vi "TOP-串口通信模块.vi"(8 "错误输入（无错误）":errorcluster, 11 "串口模块输入":T1) -> (0 "error out":errorcluster, 3 "数据输出":variant)   [LabVIEW 2017]
uses:
  be20d104-bee2-4132-b2b8-f45edb506baf.vi
  30f28544-4a48-4f37-80c2-698119a7172f.vi
  <vilib>/Instr/_visa.llb/VISA Configure Serial Port (Instr).vi
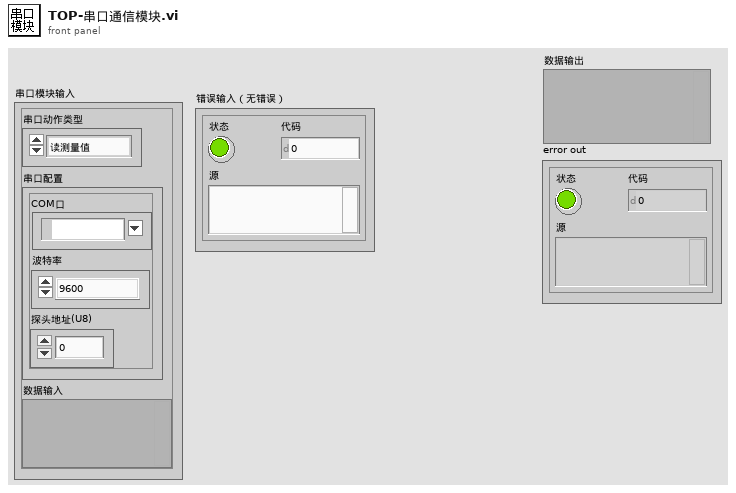
[diagram p1: front panel]
types:
  T1 = typedef "串口模块输入.ctl" = cluster{"串口动作类型":T2, "串口配置":T3, "数据输入":variant}
  T2 = typedef "串口动作类型.ctl" = enum16{"读测量值", "设置报警值", "设置地址", "设置系数", "广播修改波特率", "关闭串口"}
  T3 = typedef "串口配置.ctl" = cluster{"COM口":refnum<visa-resource-name>, "波特率":enum16{"9600", "19200"}, "探头地址(U8)":u8}
  T4 = typedef "测量值读取.ctl" = cluster{"测量值":dbl, "CRC":bool, "接收指令":string}
  T5 = typedef "探头系数.ctl" = cluster{"N1":u16, "N2":u16}
  T6 = typedef "簇-输入.ctl" = cluster{"配置文件动作":T7, "数据输入":variant}
  T7 = typedef "枚举-配置文件动作.ctl" = enum16{"初始化加载配置", "读取配置", "写入-屏幕键盘", "写入-静音延迟", "写入-主要探头类型", "写入-串口配置", "写入-累积定时", "写入-导出定时", "保存配置到文件"}
  T8 = typedef "簇-配置文件内容.ctl" = cluster{"调试模式？":bool, "屏幕键盘？":bool, "软件版本":string, "静音延迟 s":u16, "主要探头类型":T9, "串口配置":cluster{"COM口":refnum<visa-resource-name>, "波特率":enum16{"9600", "19200"}, "读写超时ms":i16, "丢包判定次数":i16}, "定时配置-累积分段":T10, "定时配置-自动导出":cluster{"定时配置-自动导出":T10, "分别导出?":bool}}
  T9 = typedef "枚举-主要探头类型.ctl" = enum16{"网络探头", "串口探头"}
  T10 = typedef "簇-定时配置.ctl" = cluster{"定时模式":enum16{"绝对时间", "相对时间"}, "单位":enum16{"年", "月", "日", "时", "分"}, "间隔":u8, "目标时刻":timestamp}
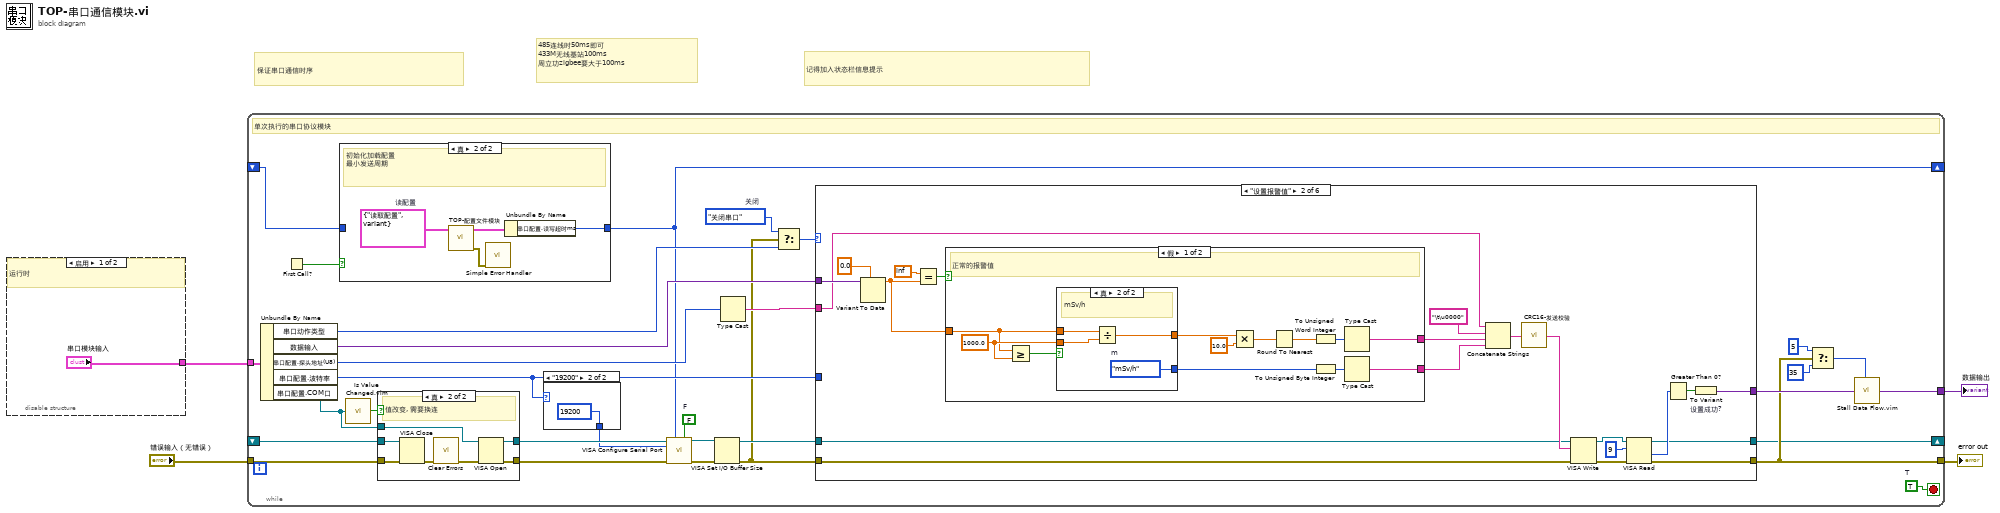
[diagram p0: block diagram]
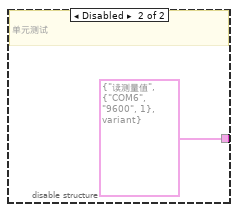
[diagram p2: hidden frame]
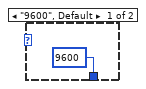
[diagram p5: hidden frame]
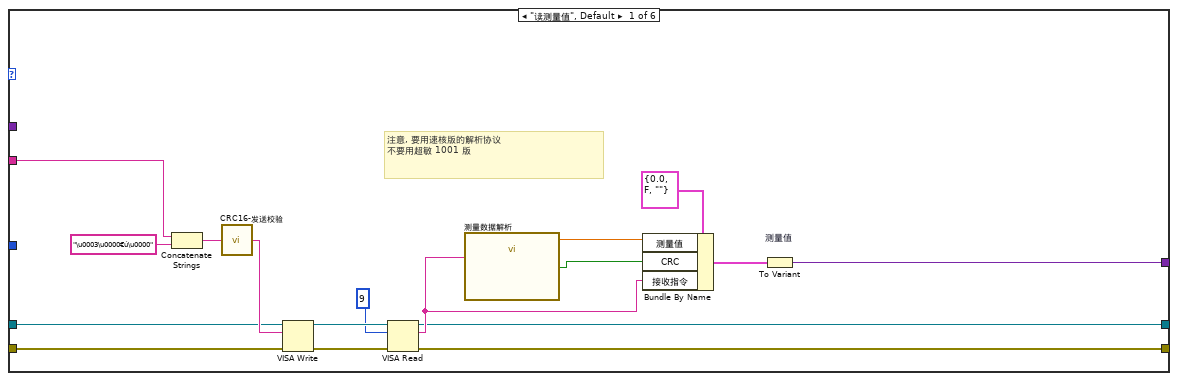
[diagram p6: hidden frame]
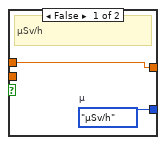
[diagram p7: hidden frame]
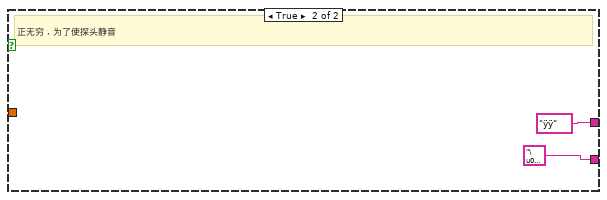
[diagram p8: hidden frame]
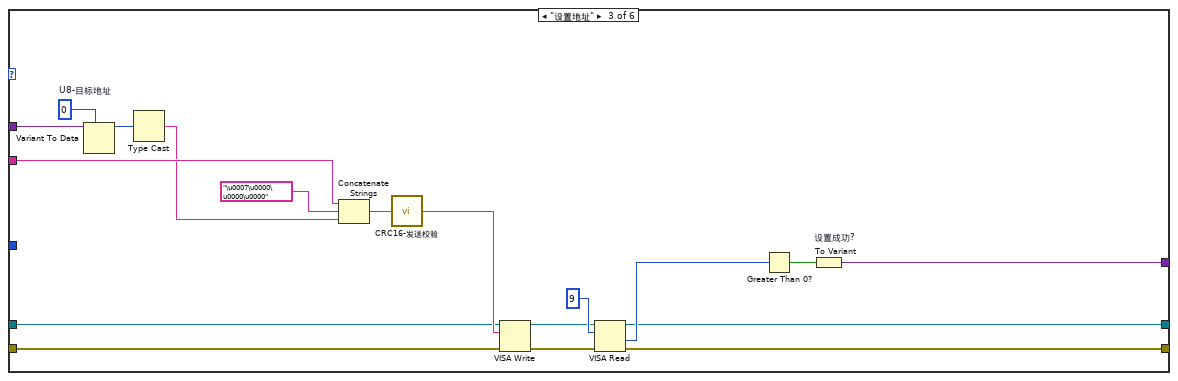
[diagram p9: hidden frame]
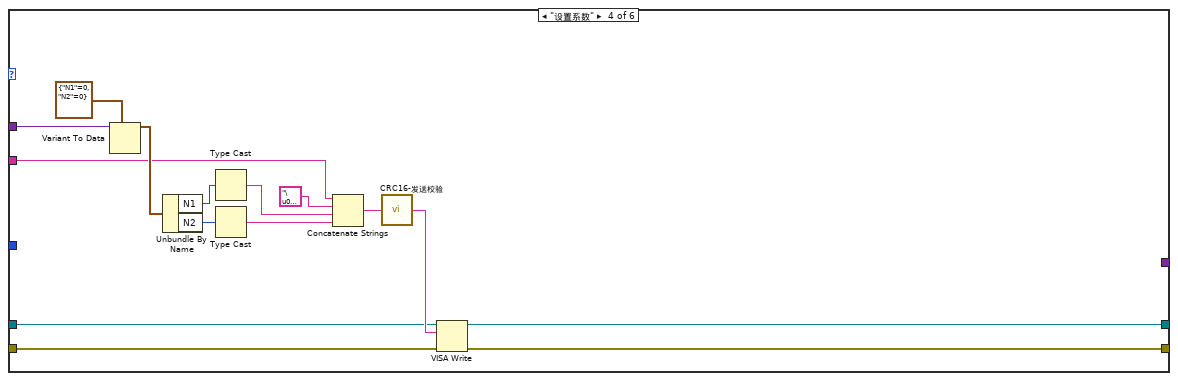
[diagram p10: hidden frame]
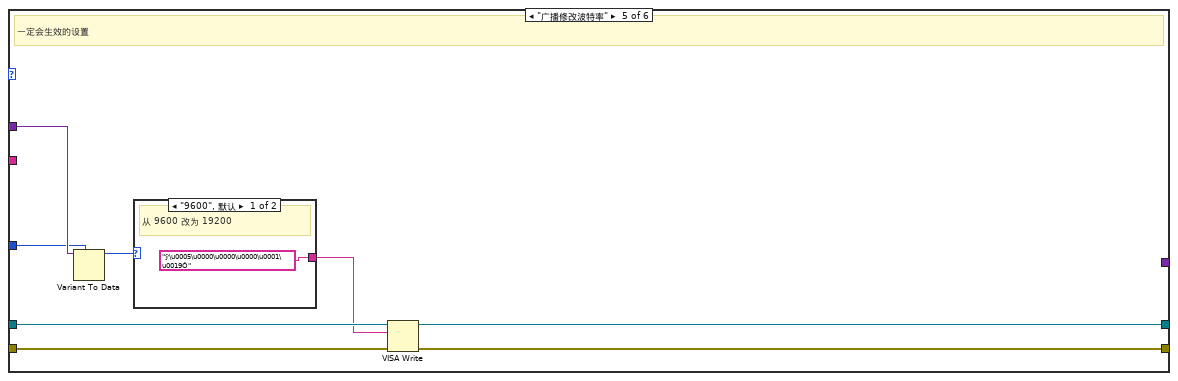
[diagram p11: hidden frame]
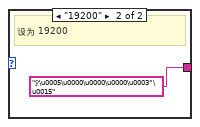
[diagram p12: hidden frame]
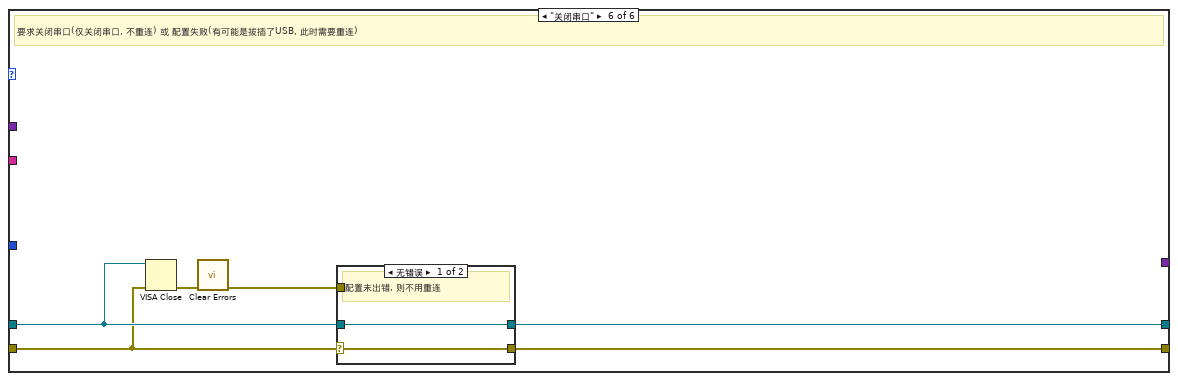
[diagram p13: hidden frame]
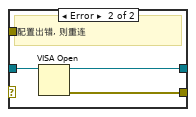
[diagram p14: hidden frame]
diagram:
  # "485连线时50ms即可\n433M无线基站100ms\n周立功zigbee要大于100ms"
  # "记得加入状态栏信息提示"
  # "保证串口通信时序"
  n1 = disable-structure shown="启用" {
    disable-tunnel: ["串口模块输入" T1 {"串口动作类型"=enum."读测量值", "串口配置"={"COM口"="COM6", "波特率"=enum."9600", "探头地址(U8)"=1}, "数据输入"=variant} ("串口模块输入")] -> w4
    frame Enabled {
      # "运行时"
    }
    frame Disabled {
      # "单元测试"
    }
  }
  n2 = while {
    tunnel: w4 -> [w36]
    tunnel: [w18] -> w3
    tunnel: "错误输入（无错误）" -> [w23]
    tunnel: [w17] -> w1
    shift-right: [w13] -> _
    shift-left: _ -> [w11]
    shift-right: [w8] -> _
    shift-left: _ -> [w7]
    stop <- w37 stop-if-true
    w22 = 串口动作类型."关闭串口"  # 关闭
    w31 = FALSE  # F
    w37 = TRUE  # T
    # "单次执行的串口协议模块"
    n3 = Unbundle By Name(w36) -> ("串口动作类型"=w21:T2, "数据输入"=w26:variant, "串口配置.探头地址(U8)"=w27:u8, "串口配置.波特率"=w25:enum16{"9600", "19200"}, "串口配置.COM口"=w12:refnum<visa-resource-name>)
    n4 = First Call?() -> (First Call?: T/F=w9:bool)
    n5 = case shown="真" w9 {
      tunnel: [w38 w39] -> w8
      tunnel: w7 -> [w38 _]
      frame False {
      }
      frame True {
        w42 = T6 {"配置文件动作"=enum."读取配置", "数据输入"=variant}  # 读配置
        # "初始化加载配置\n最小发送周期"
        n6 = call "TOP-配置文件模块.vi"("输入"=w42) -> ("error out"=w41:errorcluster, "配置文件"=w40:T8)  [unwired: 9 in]
        n7 = call <vilib>:"Simple Error Handler.vi"("error in (no error)"=w41) -> ()  [unwired: 4 in, 5 out]
        n8 = Unbundle By Name(w40) -> ("串口配置.读写超时ms"=w39:i16)
      }
    }
    n9 = call "Is Value Changed.vim"("value"=w12) -> ("changed or first call?"=w19:bool)
    n10 = case shown="真" w19 {
      tunnel: [w43 w51] -> w33
      tunnel: [w44 w50] -> w32
      tunnel: w23 -> [w43 w49]
      tunnel: w11 -> [w44 w45]
      tunnel: w12 -> [_ w46]
      frame False {
        # "值未变, 不用重连"
      }
      frame True {
        # "值改变, 需要换连"
        n11 = VISA Close(VISA resource name=w45, error in (no error)=w49) -> (error out=w48:errorcluster)
        n12 = call <vilib>:"Clear Errors.vi"("error in (no error)"=w48) -> ("error out"=w47:errorcluster)  [unwired: 5 in, 1 out]
        n13 = VISA Open(error in (no error)=w47, VISA resource name=w46) -> (VISA resource name=w50:refnum<visa-resource-name>, error out=w51:errorcluster)  [unwired: 3 out]
      }
    }
    n14 = case shown="\"19200\"" w25 {
      tunnel: [u32 9600 ("baud rate (9600)") u32 19200 ("baud rate (9600)")] -> w24
      frame "9600", Default {
      }
      frame "19200" {
      }
    }
    n15 = call-poly "VISA Configure Serial Port"("VISA resource name"=w32, "timeout (10sec)"=w8, "Enable Termination\nChar (T)"=w31, "baud rate (9600)"=w24, "error in (no error)"=w33) -> ("VISA resource name out"=w34:refnum<visa-resource-name>, "error out"=w35:errorcluster)  [unwired: 3 in, 6 out]
    n16 = VISA Set I/O Buffer Size(VISA resource name=w34, error in (no error)=w35) -> (VISA resource name out=w30:refnum<visa-resource-name>, error out=w10:errorcluster)  [unwired: 2 out]
    n17 = Type Cast(x=w27) -> (*(type *) &x=w29:string)  [unwired: 1 in]
    n18 = Select(t=w22, s=w10, f=w21) -> (s? t:f=w20:T2)
    n19 = case shown="\"设置报警值\"" w20 {
      tunnel: w26 -> [_ w85 w129 w144 w148 _]
      tunnel: w30 -> [w64 w80 w118 w133 w152 w159]
      tunnel: w29 -> [w63 w82 w125 w135 _ _]
      tunnel: [w62 w74 w115 _ _ _] -> w28
      tunnel: w25 -> [_ _ _ _ w147 _]
      tunnel: w10 -> [w61 w73 w113 w132 w150 w156]
      tunnel: [w60 w72 w114 w131 w149 w158] -> w17
      tunnel: [w54 w71 w112 w130 w145 w157] -> w13
      frame "读测量值", Default {
        # "注意, 要用速核版的解析协议\n不要用超敏 1001 版"
        n20 = Concatenate Strings(w63, "\u0003\u0000€ú\u0000") -> (w70:string)
        n21 = call "CRC16-发送校验.vi"("净数据"=w70) -> ("完整输出"=w65:string)
        n22 = VISA Write(VISA resource name=w64, write buffer=w65, error in (no error)=w61) -> (VISA resource name out=w67:refnum<visa-resource-name>, error out=w68:errorcluster)  [unwired: 1 out]
        n23 = VISA Read(VISA resource name=w67, byte count=u32 9 ("字节总数"), error in (no error)=w68) -> (VISA resource name out=w54:refnum<visa-resource-name>, read buffer=w55:string, error out=w60:errorcluster)  [unwired: 1 out]
        n24 = call "测量数据解析.vi"("完整输入"=w55) -> ("CRC？"=w58:bool, "测量值"=w57:dbl)  [unwired: 8 in, 1 out]
        n25 = Bundle By Name(cluster=T4 {"测量值"=0.0, "CRC"=FALSE, "接收指令"=""} ("测量值读取"), "测量值"=w57, "CRC"=w58, "接收指令"=w55) -> (w56:T4)
        n26 = To Variant "测量值"(anything=w56) -> (Variant=w62:variant)
      }
      frame "设置报警值" {
        n27 = Variant To Data(type=0.0, Variant=w85) -> (data=w83:dbl)  [unwired: 1 in, 1 out]
        n28 = Equal?(x=inf, y=w83) -> (x = y?=w91:bool)
        n29 = case shown="假" w91 {
          tunnel: [w94 "\u0001"] -> w88
          tunnel: [w93 "ÿÿ"] -> w89
          tunnel: w83 -> [w92 _]
          frame False {
            w102 = 1000.0 ("y")
            # "正常的报警值"
            n30 = Greater Or Equal?(x=w92, y=w102) -> (x >= y?=w103:bool)
            n31 = case shown="真" w103 {
              tunnel: w92 -> [w104 w108]
              tunnel: [w105 w109] -> w96
              tunnel: w102 -> [_ w107]
              tunnel: [w104 w106] -> w101
              frame False {
                w105 = enum8{"μSv/h", "mSv/h"}."μSv/h"  # μ
                # "μSv/h"
              }
              frame True {
                w109 = enum8{"μSv/h", "mSv/h"}."mSv/h"  # m
                # "mSv/h"
                n32 = Divide(x=w108, y=w107) -> (x/y=w106:dbl)
              }
            }
            n33 = Multiply(x=w101, y=10.0) -> (x*y=w98:dbl)
            n34 = Round To Nearest(number=w98) -> (nearest integer value=w97:dbl)
            n35 = To Unsigned Word Integer(number=w97) -> (unsigned 16bit integer=w99:u16)
            n36 = To Unsigned Byte Integer(number=w96) -> (unsigned 8bit integer=w95:u8)
            n37 = Type Cast(x=w99) -> (*(type *) &x=w93:string)  [unwired: 1 in]
            n38 = Type Cast(x=w95) -> (*(type *) &x=w94:string)  [unwired: 1 in]
          }
          frame True {
            # "正无穷 , 为了使探头静音"
          }
        }
        n39 = Concatenate Strings(w82, "\t\u0000", w89, w88) -> (w87:string)
        n40 = call "CRC16-发送校验.vi"("净数据"=w87) -> ("完整输出"=w81:string)
        n41 = VISA Write(VISA resource name=w80, write buffer=w81, error in (no error)=w73) -> (VISA resource name out=w79:refnum<visa-resource-name>, error out=w76:errorcluster)  [unwired: 1 out]
        n42 = VISA Read(VISA resource name=w79, byte count=u32 9 ("字节总数"), error in (no error)=w76) -> (VISA resource name out=w71:refnum<visa-resource-name>, return count=w77:u32, error out=w72:errorcluster)  [unwired: 1 out]
        n43 = Greater Than 0?(x=w77) -> (x > 0?=w75:bool)
        n44 = To Variant "设置成功?"(anything=w75) -> (Variant=w74:variant)
      }
      frame "设置地址" {
        w128 = u8 0  # U8-目标地址
        n45 = Variant To Data(type=w128, Variant=w129) -> (data=w127:u8)  [unwired: 1 in, 1 out]
        n46 = Type Cast(x=w127) -> (*(type *) &x=w124:string)  [unwired: 1 in]
        n47 = Concatenate Strings(w125, "\u0007\u0000\u0000\u0000", w124) -> (w123:string)
        n48 = call "CRC16-发送校验.vi"("净数据"=w123) -> ("完整输出"=w119:string)
        n49 = VISA Write(VISA resource name=w118, write buffer=w119, error in (no error)=w113) -> (VISA resource name out=w120:refnum<visa-resource-name>, error out=w122:errorcluster)  [unwired: 1 out]
        n50 = VISA Read(VISA resource name=w120, byte count=u32 9 ("字节总数"), error in (no error)=w122) -> (VISA resource name out=w112:refnum<visa-resource-name>, return count=w117:u32, error out=w114:errorcluster)  [unwired: 1 out]
        n51 = Greater Than 0?(x=w117) -> (x > 0?=w116:bool)
        n52 = To Variant "设置成功?"(anything=w116) -> (Variant=w115:variant)
      }
      frame "设置系数" {
        n53 = Variant To Data(type=T5 {"N1"=0, "N2"=0}, Variant=w144) -> (data=w142:T5)  [unwired: 1 in, 1 out]
        n54 = Unbundle By Name(w142) -> ("N1"=w137:u16, "N2"=w136:u16)
        n55 = Type Cast(x=w137) -> (*(type *) &x=w138:string)  [unwired: 1 in]
        n56 = Type Cast(x=w136) -> (*(type *) &x=w140:string)  [unwired: 1 in]
        n57 = Concatenate Strings(w135, "\u0012", w138, w140) -> (w141:string)
        n58 = call "CRC16-发送校验.vi"("净数据"=w141) -> ("完整输出"=w134:string)
        n59 = VISA Write(VISA resource name=w133, write buffer=w134, error in (no error)=w132) -> (VISA resource name out=w130:refnum<visa-resource-name>, error out=w131:errorcluster)  [unwired: 1 out]
      }
      frame "广播修改波特率" {
        # "一定会生效的设置"
        n60 = Variant To Data(type=w147, Variant=w148) -> (data=w146:enum16{"9600", "19200"})  [unwired: 1 in, 1 out]
        n61 = case shown="\"9600\", 默认" w146 {
          tunnel: ["ÿ\u0005\u0000\u0000\u0000\u0001\u0019Ô" "ÿ\u0005\u0000\u0000\u0000\u0003˜\u0015"] -> w151
          frame "9600", Default {
            # "从 9600 改为 19200"
          }
          frame "19200" {
            # "设为 19200"
          }
        }
        n62 = VISA Write(VISA resource name=w152, write buffer=w151, error in (no error)=w150) -> (VISA resource name out=w145:refnum<visa-resource-name>, error out=w149:errorcluster)  [unwired: 1 out]
      }
      frame "关闭串口" {
        # "要求关闭串口(仅关闭串口, 不重连) 或 配置失败(有可能是拔插了USB, 此时需要重连)"
        n63 = VISA Close(VISA resource name=w159, error in (no error)=w156) -> (error out=w160:errorcluster)
        n64 = call <vilib>:"Clear Errors.vi"("error in (no error)"=w160) -> ("error out"=w155:errorcluster)  [unwired: 5 in, 1 out]
        n65 = case shown="无错误" w156 {
          selector: w156 -> [w161 _]
          tunnel: w159 -> [w162 w165]
          tunnel: [w161 w164] -> w158
          tunnel: [w162 w163] -> w157
          tunnel: w155 -> [_ _]
          frame No Error {
            # "配置未出错, 则不用重连"
          }
          frame Error {
            # "配置出错, 则重连"
            n66 = VISA Open(VISA resource name=w165) -> (VISA resource name=w163:refnum<visa-resource-name>, error out=w164:errorcluster)  [unwired: 1 in, 3 out]
          }
        }
      }
    }
    n67 = Select(t=u32 5 ("milliseconds to wait"), s=w17, f=u32 35 ("milliseconds to wait")) -> (s? t:f=w14:u32)
    n68 = call "Stall Data Flow.vim"("value in"=w28, "milliseconds to wait"=w14) -> ("value out"=w18:variant)  [unwired: 1 out]
  }
  "数据输出" <- w3
  "error out" <- w1
